vi "Day 20-Parse Data.vi"(11 "Data in":string[][](array[string])) -> (2 "Input Image":bool[][](array[boolean]), 3 "Image Enhancement Lookup":bool[](array[boolean]))   [LabVIEW 2021]
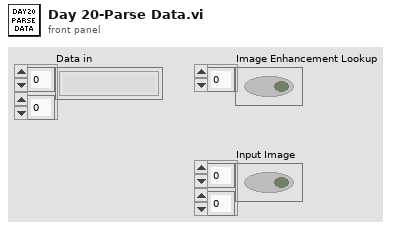
[diagram p1: front panel]
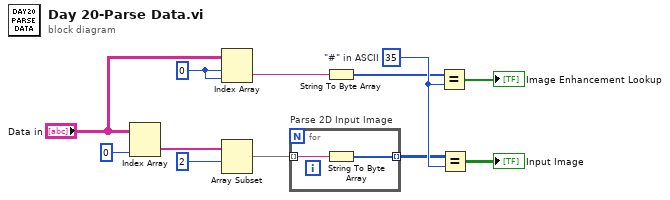
[diagram p0: block diagram]
diagram:
  w2 = 0 ("index (row)")
  w11 = u8 35  # "#" in ASCII
  n1 = Index Array(array="Data in", index (col)=0 ("disabled index (col)")) -> (element=w1:string[])  [unwired: 1 in]
  n2 = Index Array(array="Data in", index (row)=w2, index (col)=w2) -> (element=w5:string)
  n3 = Array Subset(array=w1, index=2) -> (w7:string[])  [unwired: 1 in]
  n4 = for "Parse 2D Input Image" {
    tunnel: w7 -> [w14] mode=indexing
    tunnel: [w13] -> w8 mode=indexing
    n5 = String To Byte Array(string=w14) -> (unsigned byte array=w13:u8[])
  }
  n6 = String To Byte Array(string=w5) -> (unsigned byte array=w9:u8[])
  n7 = Equal?(x=w9, y=w11) -> (x = y?=→"Image Enhancement Lookup":bool[])
  n8 = Equal?(x=w8, y=w11) -> (x = y?=→"Input Image":bool[][])
